vi "Init.vi"(8 "error in (no error)":errorcluster, 9 "View Ref":refnum<vi>, 10 "Name":string, 11 "List Box View In":refnum<class "List Box View.lvclass">) -> (0 "error out":errorcluster, 3 "List Box View Out":refnum<class "List Box View.lvclass">)   [LabVIEW 2020, in "List Box View.lvclass"]
doc: "Initializes the process and creates necessary references. Anything initialized here is released in the Clear.vi method."
uses:
  List Box View.lvclass
  View.vi
  Debug View/Debug View.lvclass
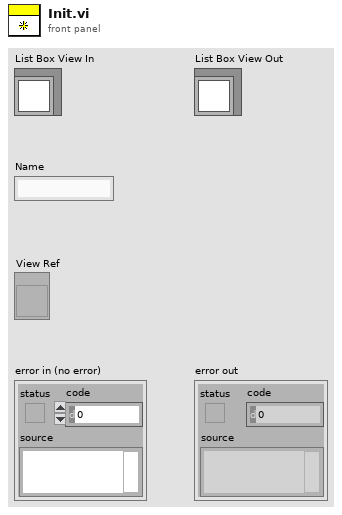
[diagram p1: front panel]
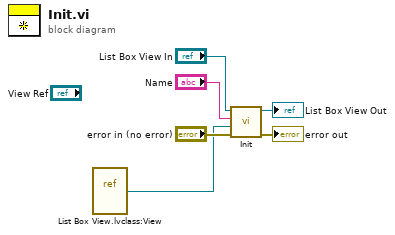
[diagram p0: block diagram]
diagram:
  n1 = vi-ref "List Box View.lvclass:View.vi"() -> (w1:refnum<vi>)
  n2 = call-parent "Init.vi"("error in (no error)"="error in (no error)", "View Ref"=w1, "Name"="Name", "Debug View In"="List Box View In") -> ("error out"=→"error out":errorcluster, "Debug View Out"=→"List Box View Out":refnum<class "List Box View.lvclass">)  [unwired: 6 in]
